vi "read term string.vi"(4 "error in (no error)":errorcluster, 6 "Termination String":string, 7 "Refnum in":refnum<k20>) -> (0 "Error Out":errorcluster, 2 "Read String":string, 3 "Reference Out":refnum<k20>)   [LabVIEW 2012]
panel:
  out "read buffer":string
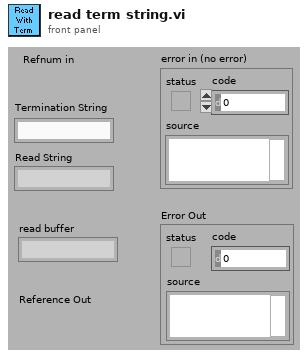
[diagram p1: front panel]
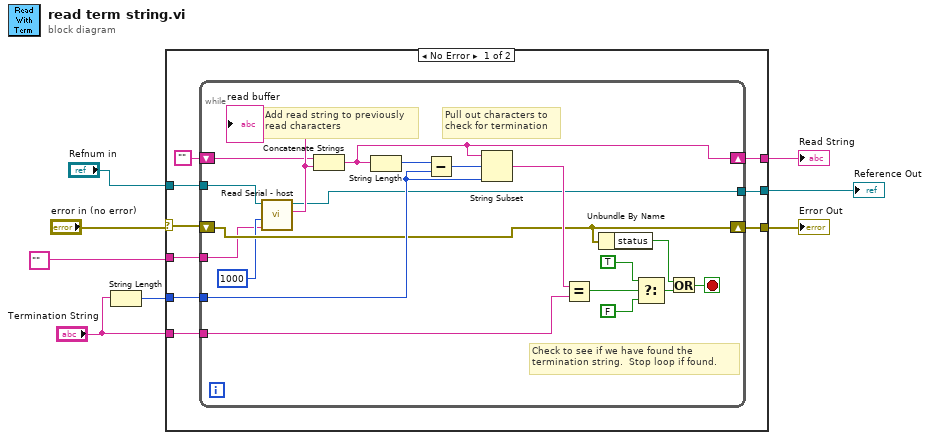
[diagram p0: block diagram]
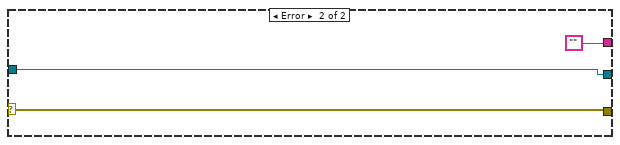
[diagram p2: hidden frame]
diagram:
  n1 = String Length(string="Termination String") -> (length=w6:i32)
  n2 = case shown="No Error" "error in (no error)" {
    selector: "error in (no error)" -> [w17 w38]
    tunnel: "Termination String" -> [w16 _]
    tunnel: w6 -> [w15 _]
    tunnel: [w13 ""] -> w5
    tunnel: [w12 w38] -> w4
    tunnel: "Refnum in" -> [w11 w37]
    tunnel: "" -> [w10 _]
    tunnel: [w9 w37] -> w1
    frame No Error {
      n3 = while {
        tunnel: w16 -> [w31]
        shift-right: [w23] -> w12
        shift-left: w17 -> [w23]
        tunnel: w15 -> [w32]
        shift-right: [w26] -> w13
        shift-left: "" -> [w35]
        tunnel: w11 -> [w21]
        tunnel: w10 -> [w19]
        tunnel: [w18] -> w9
        stop <- w25 stop-if-true
        # "Pull out characters to\ncheck for termination"
        # "Add read string to previously\nread characters"
        # "Check to see if we have found the\ntermination string.  Stop loop if found."
        n4 = call "Read Serial - host.vi"("Term Char"=w19, "Timeout (ms)"=u32 1000 ("byte count"), "Refnum in"=w21) -> ("String out"=w36:string, "Reference Out"=w18:refnum<k20>)  [unwired: 6 in, 1 out]
        "read buffer" <- w36
        n5 = Concatenate Strings(w35, w36) -> (w26:string)
        n6 = String Length(string=w26) -> (length=w34:i32)
        n7 = Subtract(x=w34, y=w32) -> (x-y=w33:i32)
        n8 = String Subset(string=w26, offset (0)=w33, length (rest)=w32) -> (substring=w27:string)
        n9 = Equal?(x=w27, y=w31) -> (x = y?=w30:bool)
        n10 = Unbundle By Name(w23) -> ("status"=w22:bool)
        n11 = Select(t=TRUE, s=w30, f=FALSE) -> (s? t:f=w24:bool)
        n12 = Or(x=w22, y=w24) -> (x .or. y?=w25:bool)
      }
    }
    frame Error {
    }
  }
  "Read String" <- w5
  "Error Out" <- w4
  "Reference Out" <- w1
